vi "zlgcan_demo_DTU.vi"() -> ()   [LabVIEW 2018]
doc: "适用的设备：CANDTU-200 XX ,CANDTU-100UR"
uses:
  data_type/ZCAN_Transmit_Data.ctl
  data_type/ZCAN_InitCAN_setting_DTU.ctl
panel:
  in  "DTU系列初始化参数":T1
  in  "开启CAN":bool
  in  "stop":bool
  in  "?":T2(tab)
  in  "CAN 通道":u32(ring) items=["0", "1"]
  in  "CAN卡型号":u32(ring)=32 items=["CANDTU-100UR"=37, "CANDTU-MINI"=33, "CANDTU-200 XX"=32, ""=0]
  in  "索引":u32(ring) items=["0", "1", "2", "3", "4", "5", "6", "7", "8"]
  in  "波特率":u32(ring)=500000 items=["1Mbps"=1000000, "800kbps"=800000, "500kbps"=500000, "250kbps"=250000, "125kbps"=125000, "100kbps"=100000, "50kbps"=50000]
  in  "自定义波特率？":bool
  in  "自定义波特率字符输入":string
  in  "工作模式":u8(ring) items=["正常", "只听"]
  in  "是否使用电阻":u8(ring)=1 items=["不使用终端电阻", "使用终端电阻"]
  out "设备句柄":u32
  out "通道句柄":u32
  out "error out":errorcluster caption="状态"
  in  "帧类型":u32(ring) items=["标准帧", "扩展帧"]
  in  "发送方式":u32(ring) items=["正常发送", "单次发送", "自发自收", "单次自发自收"]
  in  "帧格式":u32(ring) items=["数据帧", "远程帧"]
  out "数据长度":u8=8 max=8
  in  "ID":u32=18 format="0x%08x"
  in  "协议":u32(ring) items=["CAN"]
  in  "数据输入":string="11 22 33 44 55 66 77 88"
  in  "发送":bool
  in  "CAN数据帧数组":T3(array[cluster])
  out "CAN报文显示":string[][](table)
  in  "ZCAN_Transmit_Data":T4
  out "已接收帧数":u32
  # "适用的设备：CANDTU-200 XX ,CANDTU-100UR、CANDTU-MINI"
  # "停止程序前，请先关闭CAN卡"
  # "1. 确保电脑有VC++ 2005/2008/2010/2013运行库（对应32，64位）,微软常用运行库合集，点击下载（35M）。\n    http://manual.zlg.cn/Public/Uploads/2020-06-05/5ed995c271414.zip"
  # "2，如果打开设备失败，可能原因：\n（1）已经打开过一次，没有正常关闭的情况下，继续点击“打开设备”，是无法打开的。\n     需要USB重新拔插，LABVIEW重启（全部关闭），然后再“打开设备”。\n (2) 项目路径不能有中文繁体。"
  # "使用ZCANPro软件波特率计算工具计算"
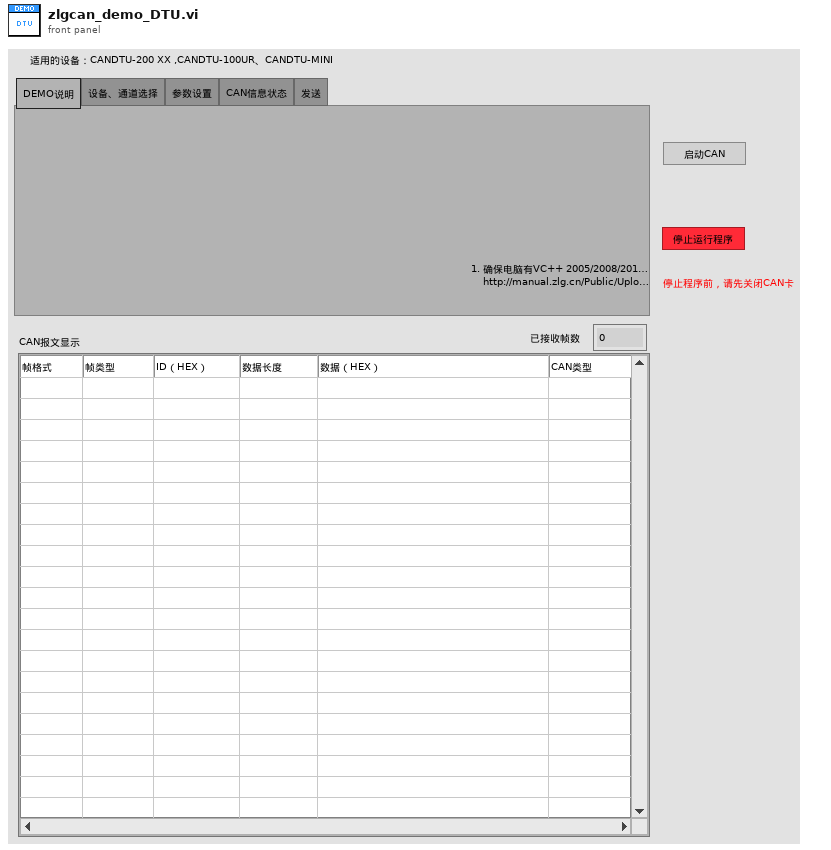
[diagram p1: front panel]
types:
  T1 = typedef "ZCAN_InitCAN_setting_DTU.ctl" = cluster{"baudrate":u32, "baud_rate_custom？":bool, "RateCustom":string, "work_mode":u32}
  T2 = enum32{"DEMO说明", "设备、通道选择", "参数设置", "CAN信息状态", "发送"}
  T3 = cluster{u32, u8, u8, u8, u8, cluster{"[0]":u8, "[1]":u8, "[2]":u8, "[3]":u8, "[4]":u8, "[5]":u8, "[6]":u8, "[7]":u8}, u64}[]
  T4 = typedef "ZCAN_Transmit_Data.ctl" = cluster{"帧类型":u32, "帧格式":u32, "ID":u32, "数据长度":u8, "DATA":cluster{"CAN数据[0]":u8, "CAN数据[1]":u8, "CAN数据[2]":u8, "CAN数据[3]":u8, "CAN数据[4]":u8, "CAN数据[5]":u8, "CAN数据[6]":u8, "CAN数据[7]":u8}, "发送方式":u32}
  T5 = cluster{"[0]":u32, "[1]":u32, "[2]":u32, "[3]":u32, "[4]":u32, "[5]":u32, "[6]":u32, "[7]":u32}
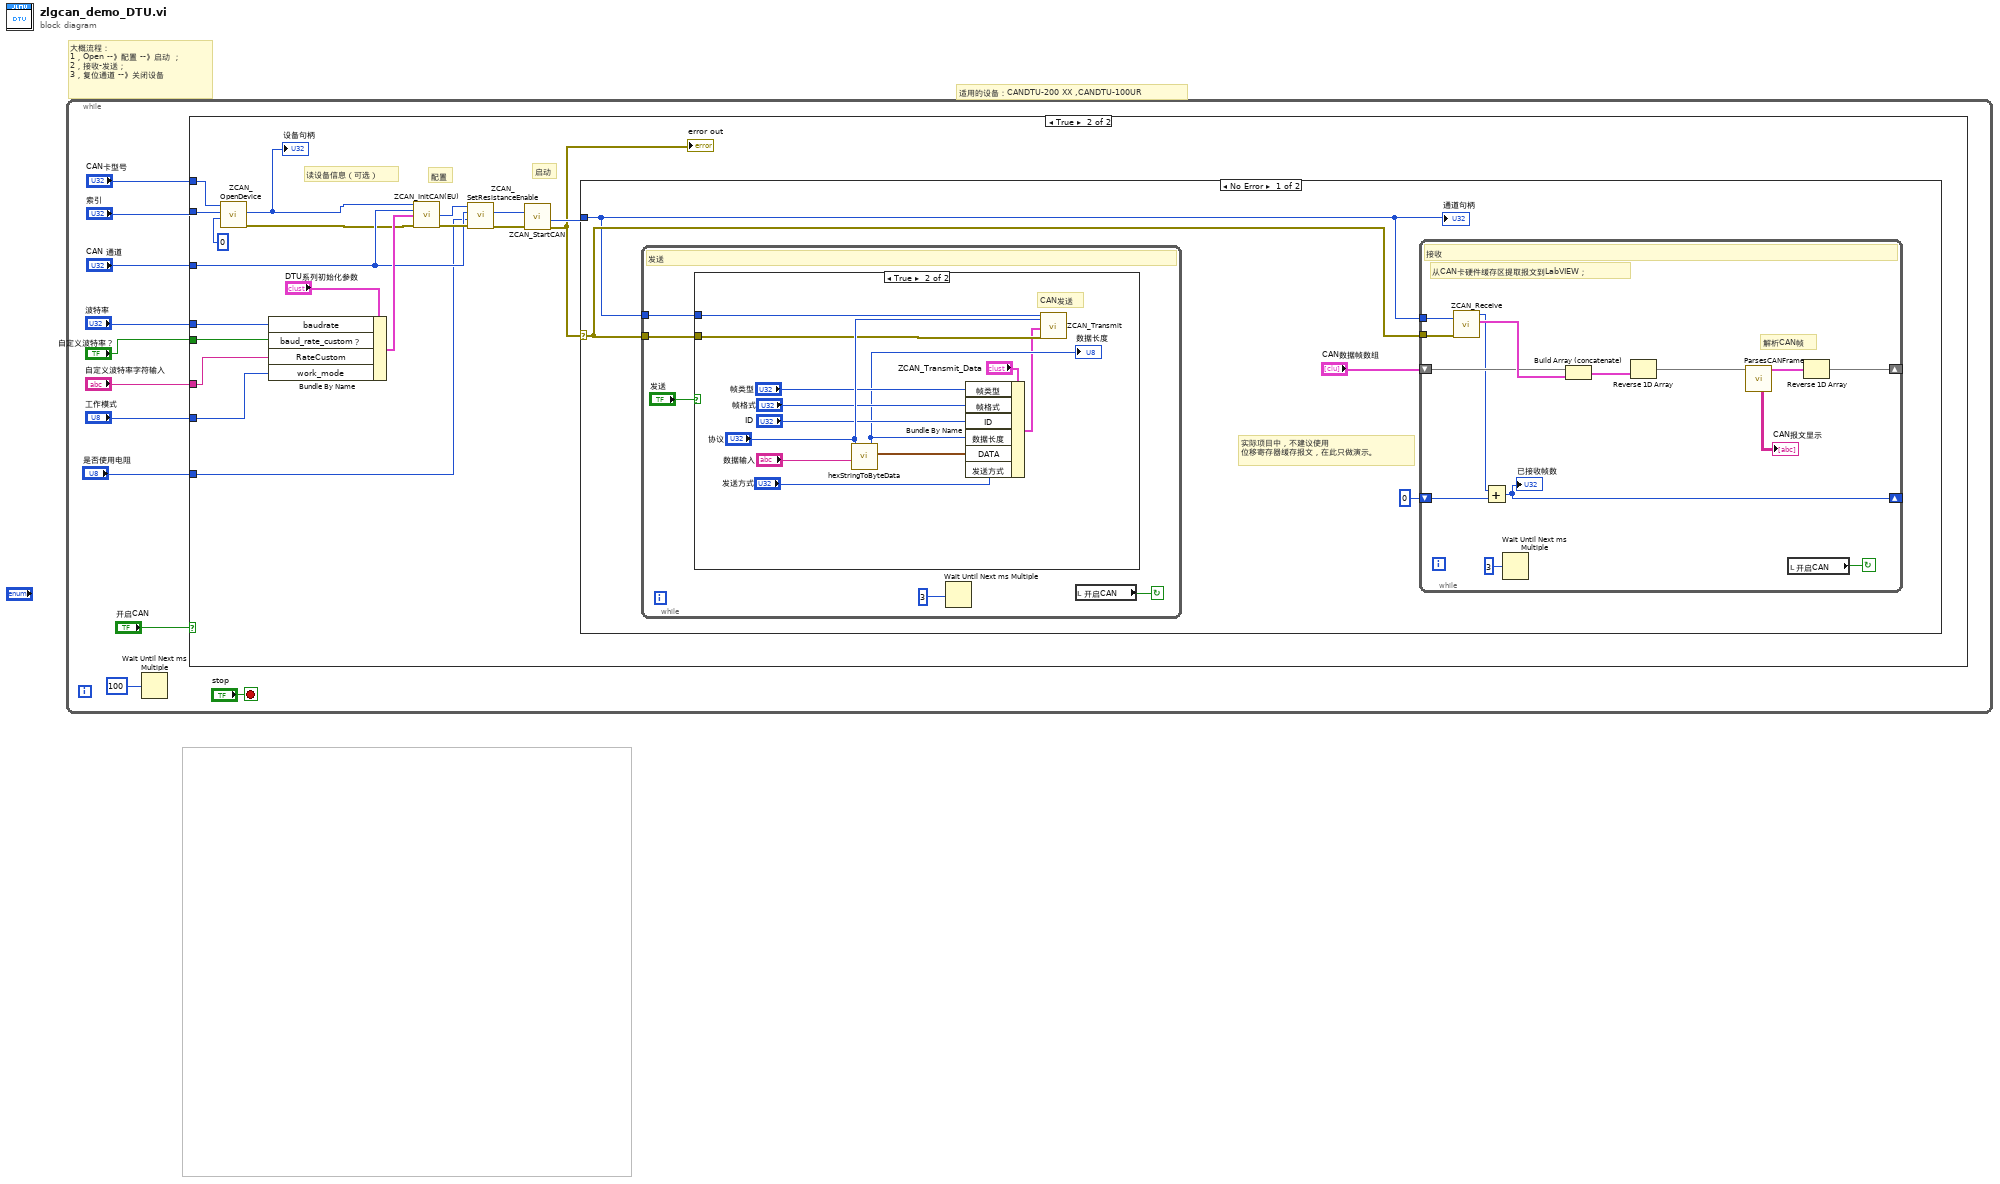
[diagram p0: block diagram]
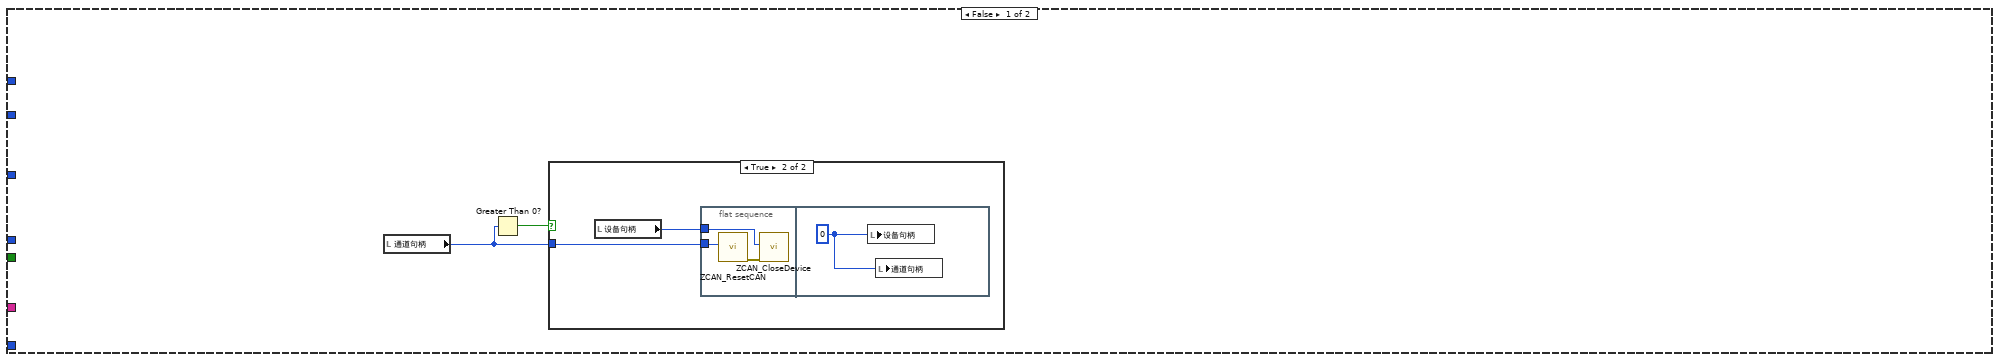
[diagram p2: hidden frame]
diagram:
  # "适用的设备：CANDTU-200 XX ,CANDTU-100UR"
  # "大概流程：\n1，Open --》配置 --》启动 ；\n2，接收-发送；\n3，复位通道 --》关闭设备"
  n1 = while {
    stop <- "stop" stop-if-true
    n2 = Wait Until Next ms Multiple(millisecond multiple=u32 100) -> ()  [unwired: 1 out]
    n3 = case shown="True" "开启CAN" {
      tunnel: "CAN 通道" -> [_ w25]
      tunnel: "CAN卡型号" -> [_ w36]
      tunnel: "索引" -> [_ w37]
      tunnel: "波特率" -> [_ w28]
      tunnel: "自定义波特率？" -> [_ w29]
      tunnel: "自定义波特率字符输入" -> [_ w30]
      tunnel: "工作模式" -> [_ w31]
      tunnel: "是否使用电阻" -> [_ w24]
      frame False {
        # "关闭CAN卡"
        n4 = local read "通道句柄"() -> (w12:u32)
        n5 = Greater Than 0?(x=w12) -> (x > 0?=w13:bool)
        n6 = case shown="True" w13 {
          tunnel: w12 -> [_ w15]
          frame False {
          }
          frame True {
            n7 = local read "设备句柄"() -> (w14:u32)
            n8 = flat-sequence {
              tunnel: w15 -> [w17]
              tunnel: w14 -> [w16]
              frame #0 {
                n9 = call "ZCAN_ResetCAN.vi"("can_handle"=w17) -> ("error out"=w18:errorcluster)  [unwired: 9 in, 1 out]
                n10 = call "ZCAN_CloseDevice.vi"("error in (no error)"=w18, "device_handle"=w16) -> ()  [unwired: 8 in, 2 out]
              }
              frame #1 {
                w19 = u32 0 ("can_index_handle(out)")
                n11 = local write "设备句柄"(w19) -> ()
                n12 = local write "通道句柄"(w19) -> ()
              }
            }
          }
        }
      }
      frame True {
        # "启动"
        # "配置"
        # "读设备信息（可选）"
        n13 = call "ZCAN_OpenDevice.vi"("reserved"=0, "device_index"=w37, "device_type"=w36) -> ("error out"=w20:errorcluster, "DEVICE_HANDLE"=w21:u32)  [unwired: 7 in]
        "设备句柄" <- w21
        n14 = Bundle By Name(cluster="DTU系列初始化参数", "baudrate"=w28, "baud_rate_custom？"=w29, "RateCustom"=w30, "work_mode"=w31) -> (w33:T1)
        n15 = call "ZCAN_InitCAN(EU).vi"("device_hande"=w21, "can_index"=w25, "ZCAN_InitCAN_Setting_EU"=w33, "error in (no error)"=w20) -> ("can_index_handle"=w23:u32, "error out"=w27:errorcluster)  [unwired: 10 in]
        n16 = call "ZCAN_SetResistanceEnable.vi"("error in (no error)"=w27, "enable"=w24, "can_index"=w25, "can_index_handle"=w23) -> ("error out"=w26:errorcluster, "can_index_handle(out)"=w22:u32)  [unwired: 6 in]
        n17 = call "ZCAN_StartCAN.vi"("error in (no error)"=w26, "can_index_handle"=w22) -> ("error out"=w34:errorcluster, "can_index_handle(out)"=w35:u32)  [unwired: 7 in, 1 out]
        "error out" <- w34
        n18 = case shown="No Error" w34 {
          selector: w34 -> [w41 _]
          tunnel: w35 -> [w40 _]
          frame No Error {
            # "实际项目中，不建议使用\n位移寄存器缓存报文，在此只做演示。"
            n19 = while {
              tunnel: w40 -> [w59]
              tunnel: w41 -> [w57]
              stop <- w58 continue-if-true
              # "发送"
              n20 = case shown="True" "发送" {
                tunnel: w59 -> [_ w66]
                tunnel: w57 -> [_ w67]
                frame False {
                }
                frame True {
                  # "CAN发送"
                  n21 = call "hexStringToByteData.vi"("数据输入"="数据输入", "协议"="协议") -> ("CAN_data"=w63:T5, "字节数"=w68:i32)  [unwired: 7 in, 1 out]
                  "数据长度" <- w68
                  n22 = Bundle By Name(cluster="ZCAN_Transmit_Data", "帧类型"="帧类型", "帧格式"="帧格式", "ID"="ID", "数据长度"=w68, "DATA"=w63, "发送方式"="发送方式") -> (w62:T4)
                  n23 = call "ZCAN_Transmit.vi"("can_index_handle"=w66, "协议"="协议", "ZCAN_Transmit_Data"=w62, "error in (no error)"=w67) -> ()  [unwired: 15 in, 1 out]
                }
              }
              n24 = Wait Until Next ms Multiple(millisecond multiple=u32 3) -> ()  [unwired: 1 out]
              n25 = local read "开启CAN"() -> (w58:bool)
            }
            n26 = while {
              tunnel: w41 -> [w54]
              tunnel: w40 -> [w53]
              shift-right: [w55] -> _
              shift-left: 0 -> [w44]
              shift-right: [w47] -> _
              shift-left: "CAN数据帧数组" -> [w50]
              stop <- w52 continue-if-true
              # "从CAN卡硬件缓存区提取报文到LabVIEW；"
              # "解析CAN帧"
              # "接收"
              n27 = call "ZCAN_Receive.vi"("error in (no error)"=w54, "can_handle"=w53) -> ("CAN数据帧数组"=w51:T3, "Receive_Num"=w45:u32)  [unwired: 2 in, 2 out]
              n28 = Add(x=w45, y=w44) -> (x+y=w55:u32)
              "已接收帧数" <- w55
              n29 = Wait Until Next ms Multiple(millisecond multiple=u32 3) -> ()  [unwired: 1 out]
              n30 = Build Array (concatenate)(w50, w51) -> (w49:T3)
              n31 = Reverse 1D Array(array=w49) -> (reversed array=w46:T3)
              n32 = call "ParsesCANFrame.vi"("CAN数据帧数组"=w46) -> ("CAN数据帧数组(out)"=w48:T3, "CAN报文显示"=→"CAN报文显示":string[][])  [unwired: 9 in]
              n33 = local read "开启CAN"() -> (w52:bool)
              n34 = Reverse 1D Array(array=w48) -> (reversed array=w47:T3)
            }
            "通道句柄" <- w40
          }
          frame Error {
          }
        }
      }
    }
  }
